vi "subDisableArray.vi"(0 "Array":refnum<vi>[](array[refnum]), 1 "Enable":bool) -> ()   [LabVIEW 2020]
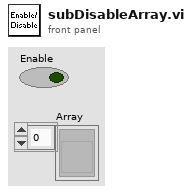
[diagram p1: front panel]
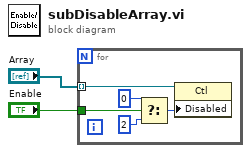
[diagram p0: block diagram]
diagram:
  n1 = for {
    tunnel: "Array" -> [w7] mode=indexing
    tunnel: "Enable" -> [w5]
    n2 = Select(t=0, s=w5, f=2) -> (s? t:f=w6:i32)
    n3 = property class="Ctl"(reference=w7, "Disabled"=w6) -> ()  [unwired: 1 in, 2 out]
  }
